vi "Create SingleFileCopy Job.vi"(5 "Job.SingleFileCopy in":refnum<class "Job.SingleFileCopy.lvclass">, 6 "JobReport type":refnum<class "JobReport.lvclass">, 7 "Job Name":string, 8 "error in (no error)":errorcluster, 10 "Destination":path, 11 "Source":path) -> (0 "error out":errorcluster, 3 "Job.SingleFileCopy":refnum<class "Job.SingleFileCopy.lvclass">)   [LabVIEW 2013, in "Job.SingleFileCopy.lvclass"]
uses:
  Job.SingleFileCopy.lvclass
  <vilib>/LabVIEW Open Source Project/Cron Scheduler/JobReport/JobReport.lvclass
  Job.SingleFileCopy.lvclass/Job.SingleFileCopy.ctl
  <vilib>/LabVIEW Open Source Project/Cron Scheduler/Job/Job.lvclass
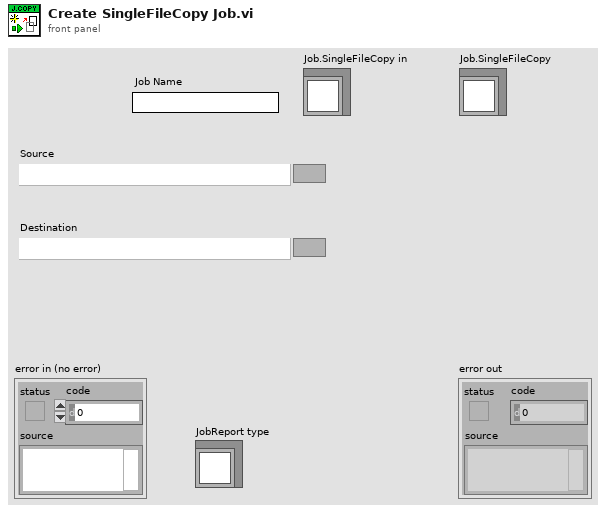
[diagram p1: front panel]
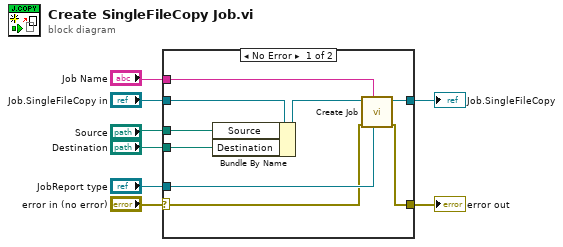
[diagram p0: block diagram]
diagram:
  n1 = case shown="No Error" "error in (no error)" {
    selector: "error in (no error)" -> [w12 w19]
    tunnel: [w11 w19] -> w7
    tunnel: [w15 w18] -> w5
    tunnel: "Job.SingleFileCopy in" -> [w17 w18]
    tunnel: "Job Name" -> [w14 _]
    tunnel: "JobReport type" -> [w13 _]
    tunnel: "Destination" -> [w10 _]
    tunnel: "Source" -> [w9 _]
    frame No Error {
      n2 = Bundle By Name(cluster=w17, "Source"=w9, "Destination"=w10) -> (w16:refnum<class "Job.SingleFileCopy.lvclass">)
      n3 = call <vilib>:"Create Job.vi"("JobReport type"=w13, "Job Name"=w14, "error in (no error)"=w12, "Job in"=w16) -> ("error out"=w11:errorcluster, "Job"=w15:refnum<class "Job.SingleFileCopy.lvclass">)  [unwired: 6 in]
    }
    frame Error {
    }
  }
  "error out" <- w7
  "Job.SingleFileCopy" <- w5
